vi "Read Configuration API.vi"   [LabVIEW 2019, in "Architecture.lvlib"]
uses:
  Architecture.lvlib
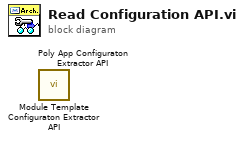
[diagram p0: block diagram]
diagram:
  n1 = call "Module Template Configuraton Extractor API.vi"() -> ()  [unwired: 10 in, 2 out]
  n2 = call "Poly App Configuraton Extractor API.vi"() -> ()  [unwired: 10 in, 2 out]
